vi "Check Output For Octave Errors.vi"(8 "error in":errorcluster, 10 "read buffer":string) -> (0 "error out":errorcluster)   [LabVIEW 2013, in "GOLPI library.lvlib"]
doc: "Parse stdout output of GNU Octave and search for GNU Octave errors. If any found, generates LabVIEW error.\n\n---\nGOLPI works only with lv_pro.dll library, which is part of vipm package or should be delivered together with packed library. Placement of this dll is selected in terminal of Start GNU Octave.vi."
uses:
  GOLPI library.lvlib
  Private/Type Definitions/Custom Error Codes Enum Type Def.vi
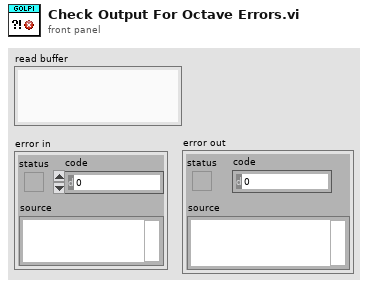
[diagram p1: front panel]
types:
  T1 = typedef "GOLPI library.lvlib/Custom Error Codes Enum Type Def.vi" = enum16{"no error", "00 working directory PAR1 missing", "01 octave binary PAR1 missing", "02 octave report error PAR1", "03 empty output last cmd PAR1", "04 missing temporary file PAR1", "05 pwd PAR 1 not exist", "06 oct package not installed", "10 var PAR1 not string, vect", "11 var PAR1 not num, scal, ~compl", "12 var PAR1 not num, scal, compl", "13 var PAR1 not num, vect, ~compl", "14 var PAR1 not num, vect, compl", "15 var PAR1 not num, mat, ~compl", "16 var PAR1 not num, mat, ~compl", "30 read timeout", "60 bitstream transport failed", "61 bitstream decode error PAR1", "62 bitstream cannot be set", "70 struct transfer not possible", "80 struct: cluster elem. PAR1 not implem.", "81 struct: structure field PAR1 not implem.", "82 struct: size mismatch of PAR1", "83 struct: type mismatch of PAR1", "98 internal error", "99 not finished", "90 Not supported in Matlab mode", "91 Matlab variable transfer error", "92 Matlab Script Error"}
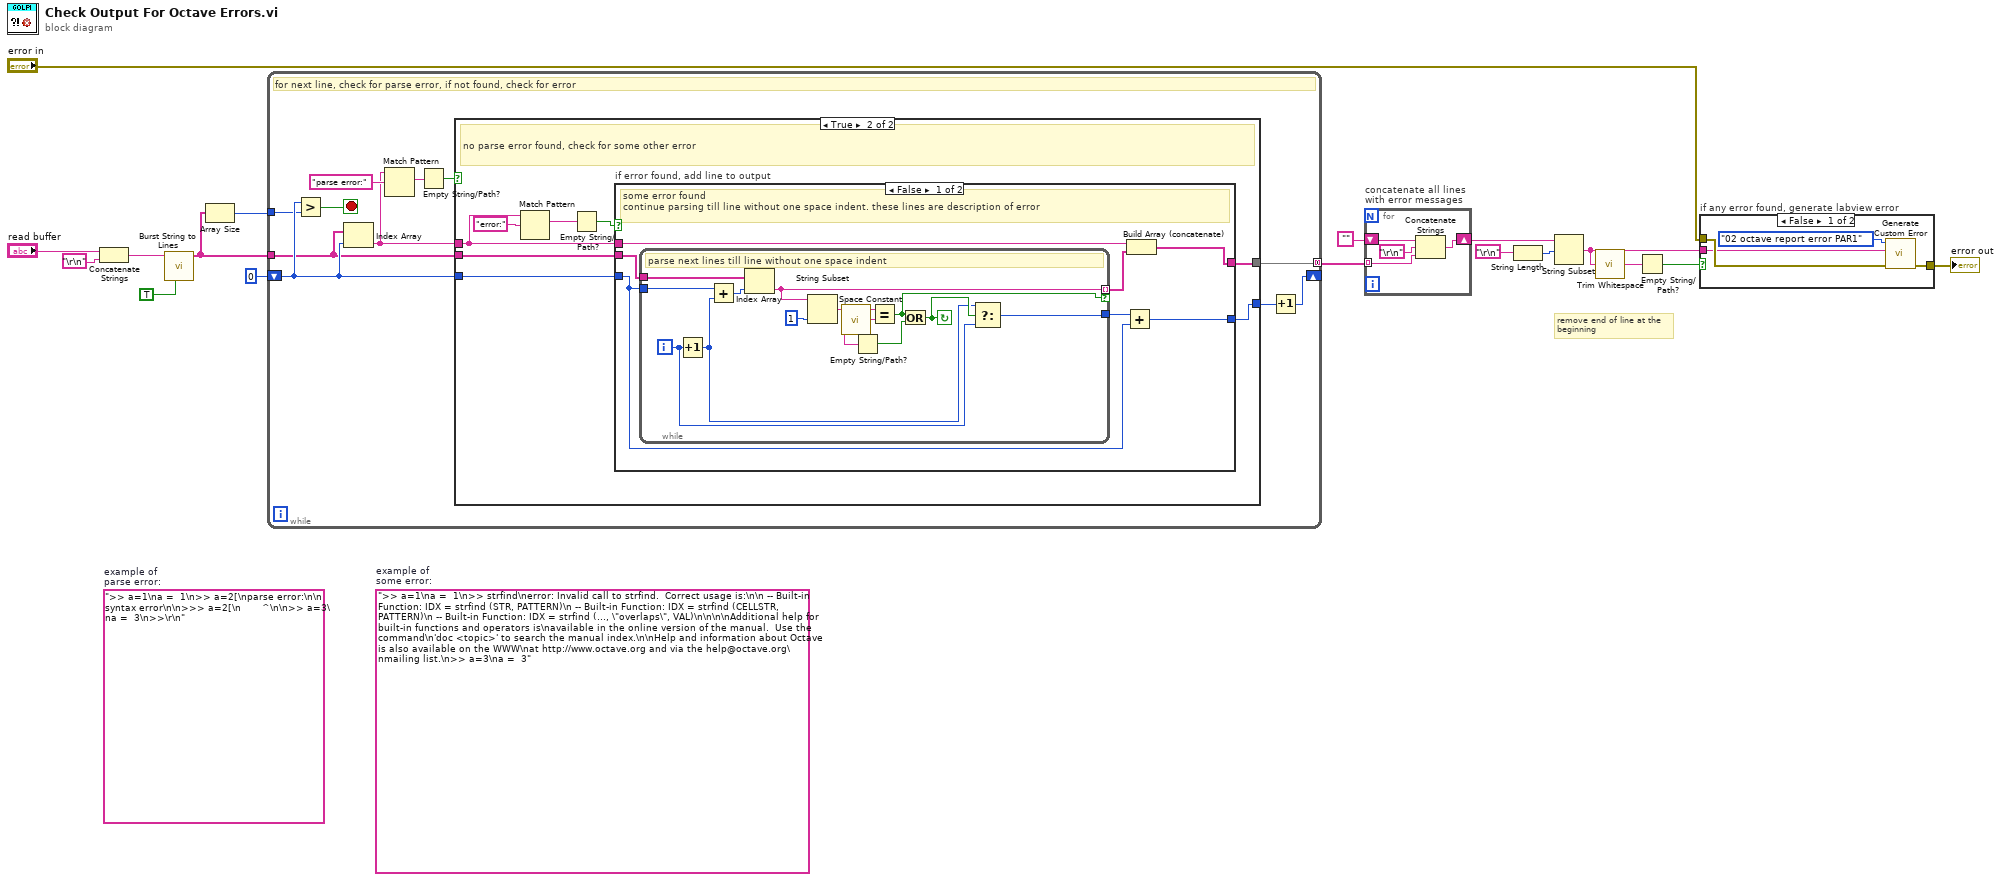
[diagram p0: block diagram]
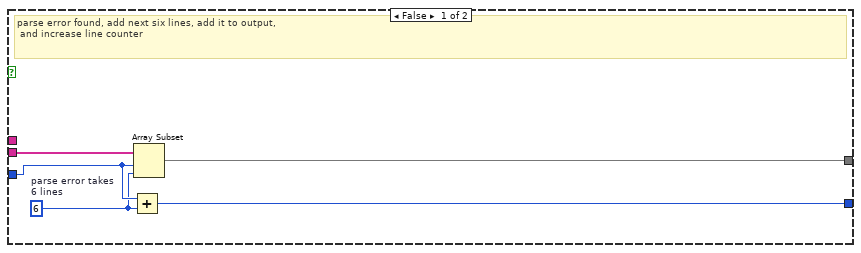
[diagram p2: hidden frame]
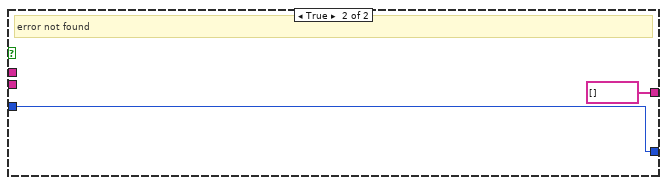
[diagram p3: hidden frame]
diagram:
  (unwired) ">> a=1\na =  1\n>> strfind\nerror: Invalid call to strfind.  Correct usage is:\n\n -- Built-in Function: IDX = strfind (STR, PATTERN)\n -- Built-in Function: IDX = strfind (CELLSTR, PATTERN)\n -- Built-in Function: IDX = strfind (..., \"overlaps\", VAL)\n\n\n\nAdditional help for built-in functions and operators is\navailable in the online version of the manual.  Use the command\n'doc <topic>' to search the manual index.\n\nHelp and information about Octave is also available on the WWW\nat http://www.octave.org and via the help@octave.org\nmailing list.\n>> a=3\na =  3"  # example of some error:
  (unwired) ">> a=1\na =  1\n>> a=2[\nparse error:\n\n  syntax error\n\n>>> a=2[\n       ^\n\n>> a=3\na =  3\n>>\r\n"  # example of parse error:
  # "remove end of line at the\nbeginning"
  n1 = Concatenate Strings("read buffer", "\r\n") -> (w3:string)
  n2 = call "Burst String to Lines.vi"("preserve leading spaces"=TRUE, "read buffer"=w3) -> ("lines"=w2:string[])  [unwired: 9 in]
  n3 = Array Size(array=w2) -> (size(s)=w8:i32)
  n4 = while {
    shift-right: [w20] -> _
    shift-left: 0 ("index") -> [w24]
    tunnel: [w25] -> w10 mode=concatenating
    tunnel: w8 -> [w23]
    tunnel: w2 -> [w19]
    stop <- w22 stop-if-true
    # "for next line, check for parse error, if not found, check for error"
    n5 = Greater?(x=w24, y=w23) -> (0:w22:bool)
    n6 = Index Array(array=w19, index=w24) -> (element=w18:string)
    n7 = Match Pattern(string=w18, regular expression="parse error:") -> (match substring=w27:string)  [unwired: 1 in, 3 out]
    n8 = Empty String/Path?(string/path=w27) -> (empty?=w26:bool)
    n9 = case shown="True" w26 {
      tunnel: w19 -> [w32 w36]
      tunnel: w24 -> [w31 w35]
      tunnel: [w29 w38] -> w25
      tunnel: [w33 w34] -> w21
      tunnel: w18 -> [_ w37]
      frame False {
        w30 = 6  # parse error takes 6 lines
        # "parse error found, add next six lines, add it to output,\n and increase line counter"
        n10 = Add(x=w31, y=w30) -> (x+y=w33:i32)
        n11 = Array Subset(array=w32, index=w31, length=w30) -> (w29:string[])
      }
      frame True {
        # "no parse error found, check for some other error"
        n12 = Match Pattern(string=w37, regular expression="error:") -> (match substring=w41:string)  [unwired: 1 in, 3 out]
        n13 = Empty String/Path?(string/path=w41) -> (empty?=w39:bool)
        n14 = case "if error found, add line to output" shown="False" w39 {
          tunnel: [w47 string[] []] -> w38
          tunnel: w37 -> [w48 _]
          tunnel: w36 -> [w46 _]
          tunnel: w35 -> [w43 w62]
          tunnel: [w42 w62] -> w34
          frame False {
            # "some error found\ncontinue parsing till line without one space indent. these lines are description of error"
            n15 = while {
              tunnel: w46 -> [w61]
              tunnel: w43 -> [w60]
              tunnel: [w54] -> w45 mode=indexing if=w49
              tunnel: [w50] -> w44
              i -> [w51]
              stop <- w53 continue-if-true
              # "parse next lines till line without one space indent"
              n16 = Increment(x=w51) -> (x+1=w52:i32)
              n17 = Add(x=w60, y=w52) -> (x+y=w59:i32)
              n18 = Index Array(array=w61, index=w59) -> (element=w54:string)
              n19 = String Subset(string=w54, length (rest)=1 ("length (rest)")) -> (substring=w56:string)  [unwired: 1 in]
              n20 = call <vilib>:"Space Constant.vi"() -> ("String"=w57:string)
              n21 = Empty String/Path?(string/path=w56) -> (empty?=w55:bool)
              n22 = Equal?(x=w56, y=w57) -> (x = y?=w49:bool)
              n23 = Or(x=w49, y=w55) -> (x .or. y?=w53:bool)
              n24 = Select(t=w52, s=w53, f=w51) -> (s? t:f=w50:i32)
            }
            n25 = Add(x=w44, y=w43) -> (x+y=w42:i32)
            n26 = Build Array (concatenate)(w48, w45) -> (w47:string[])
          }
          frame True {
            # "error not found"
          }
        }
      }
    }
    n27 = Increment(x=w21) -> (x+1=w20:i32)
  }
  n28 = for "concatenate all lines\nwith error messages" {
    tunnel: w10 -> [w65] mode=indexing
    shift-right: [w67] -> w7
    shift-left: "" -> [w64]
    n29 = Concatenate Strings(w64, "\r\n", w65) -> (w67:string)
  }
  n30 = String Length(string="\r\n") -> (length=w4:i32)
  n31 = String Subset(string=w7, offset (0)=w4) -> (substring=w6:string)  [unwired: 1 in]
  n32 = call <vilib>:"Trim Whitespace.vi"("string"=w6) -> ("trimmed string"=w12:string)  [unwired: 1 in]
  n33 = Empty String/Path?(string/path=w12) -> (empty?=w17:bool)
  n34 = case "if any error found, generate labview error" shown="False" w17 {
    tunnel: w6 -> [w68 _]
    tunnel: "error in" -> [w71 w72]
    tunnel: [w70 w72] -> w15
    frame False {
      n35 = call "Generate Custom Error.vi"("error in"=w71, "PAR1"=w68, "GOLPI error"=Custom_Error_Codes_Enum_Type_Def.vi."02 octave report error PAR1" ("Enum")) -> ("error out"=w70:errorcluster)  [unwired: 8 in]
    }
    frame True {
    }
  }
  "error out" <- w15
